vi "niDDC template.vi"(8 "error in (no error)":errorcluster, 11 "Class in":refnum<class "7976R_v1.lvclass">) -> (0 "error out":errorcluster, 3 "Class out":refnum<class "7976R_v1.lvclass">)   [LabVIEW 2015, in "7976R_v1.lvclass"]
uses:
  <userlib>/SE-APP-Receiver/NI5772/7976R_v1/7976R_v1.lvclass
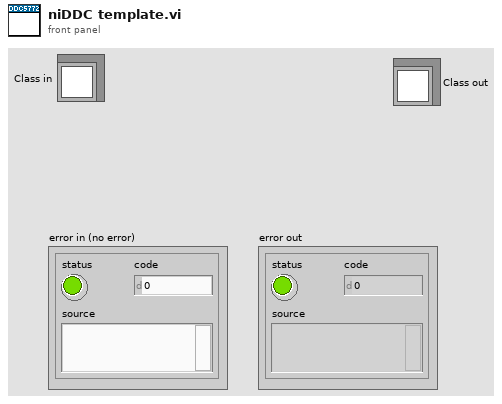
[diagram p1: front panel]
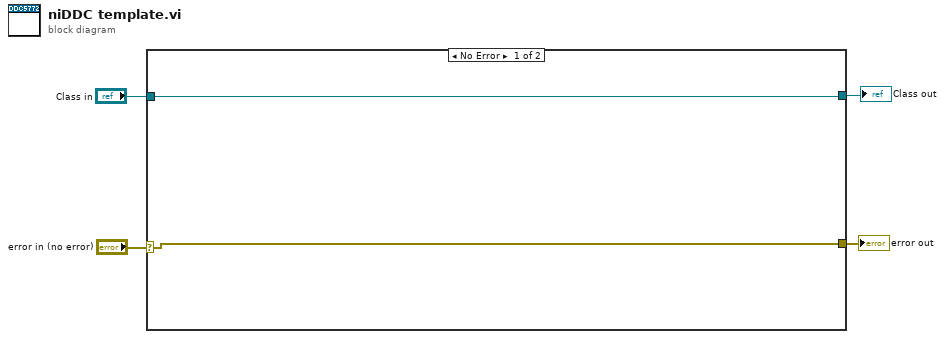
[diagram p0: block diagram]
diagram:
  n1 = case shown="No Error" "error in (no error)" {
    selector: "error in (no error)" -> [w5 w8]
    tunnel: [w5 w8] -> w4
    tunnel: "Class in" -> [w6 w7]
    tunnel: [w6 w7] -> w1
    frame No Error {
    }
    frame Error {
    }
  }
  "error out" <- w4
  "Class out" <- w1
